vi "Lookup Services of Type.vi"(7 "Type":refnum<class>, 8 "error in (no error)":errorcluster, 11 "Service Container in":refnum<class "Service Container.lvclass">) -> (0 "error out":errorcluster, 2 "Services":refnum<class "Service.lvclass">[](array[class]), 3 "Service Container out":refnum<class "Service Container.lvclass">)   [LabVIEW 2020, in "Vecto.lvlib" / "Service Container.lvclass"]
uses:
  Service Container.lvclass
  Service/Service.lvclass
  Service Container.lvclass/Service Container.ctl
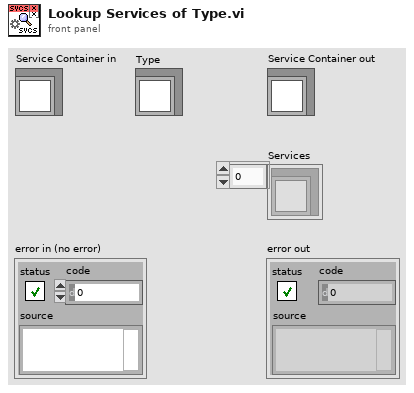
[diagram p1: front panel]
types:
  T1 = typedef "Vecto.lvlib/Service Container.lvclass/Services.ctl" = map{string, map{string, refnum<class "Service.lvclass">}}
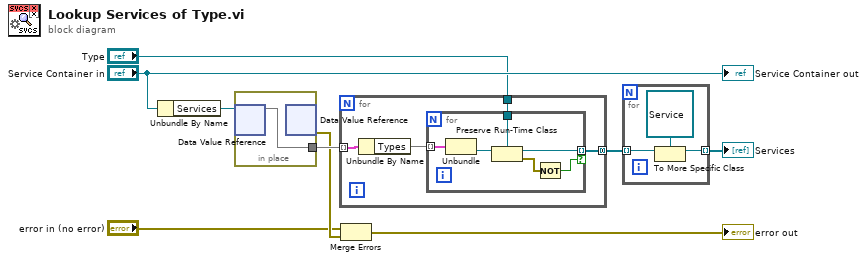
[diagram p0: block diagram]
diagram:
  n1 = Unbundle By Name("Service Container in") -> ("Services"=w9:refnum<data-value>)
  n2 = in-place {
    in-place-border: [w10] -> w7
    n3 = in-place-dvr #1(w9) -> (w10:T1)  [unwired: 1 out]
    n4 = in-place-dvr #1() -> (w5:errorcluster)  [unwired: 1 in, 1 out]
  }
  n5 = for {
    tunnel: w7 -> [w14] mode=indexing
    tunnel: "Type" -> [w12]
    tunnel: [w11] -> w2 mode=concatenating
    n6 = Unbundle By Name(w14) -> ("Types"=w13:map{string, refnum<class "Service.lvclass">})
    n7 = for {
      tunnel: w13 -> [w20] mode=indexing
      tunnel: w12 -> [w18]
      tunnel: [w17] -> w11 mode=indexing if=w15
      n8 = Unbundle(w20) -> ("Service"=w19:refnum<class "Service.lvclass">)  [unwired: 1 out]
      n9 = Preserve Run-Time Class(object in=w19, 2:w18) -> (object out=w17:refnum<class>, error out=w16:errorcluster)  [unwired: 1 in]
      n10 = Not(x=w16) -> (.not. x?=w15:bool)
    }
  }
  n11 = Merge Errors("error in (no error)", w5) -> (→"error out":errorcluster)
  n12 = for {
    tunnel: w2 -> [w23] mode=indexing
    tunnel: [w21] -> w1 mode=indexing
    n13 = To More Specific Class(target class=refnum<class "Service.lvclass"> refnum ("Vecto.lvlib:Service.lvclass"), reference=w23) -> (specific class reference=w21:refnum<class "Service.lvclass">)  [unwired: 1 in, 1 out]
  }
  "Services" <- w1
  "Service Container out" <- "Service Container in"
